vi "Read 3D Quiver  Property Array.vi"(8 "error in (no error)":errorcluster, 11 "3D Quiver.lvclass in":refnum<class "3D Quiver.lvclass">) -> (0 "error out":errorcluster, 2 "3D Quiver Property Array":T1, 3 "3D Quiver.lvclass out":refnum<class "3D Quiver.lvclass">)   [LabVIEW 2020, in "3D Quiver.lvclass"]
uses:
  <vilib>/Math Plots/3D Math Plots/3D Quiver/3D Quiver/3D Quiver.lvclass
  <vilib>/Math Plots/3D Math Plots/3D Quiver/3D Quiver/Typedef/3D Quiver Property Array.ctl
  <vilib>/Math Plots/3D Math Plots/3D Quiver/3D Quiver/Typedef/3D Quiver Property.ctl
  <vilib>/Math Plots/3D Math Plots/3D Plot/3D Plot/Typedef/Line Type.ctl
  <vilib>/Math Plots/3D Math Plots/3D Plot/3D Plot/Typedef/Color Ramp Cluster.ctl
  <vilib>/Math Plots/3D Math Plots/3D Quiver/3D Quiver/3D Quiver.lvclass/3D Quiver.ctl
  <vilib>/Math Plots/3D Math Plots/3D Plot/3D Plot/3D Plot.lvclass
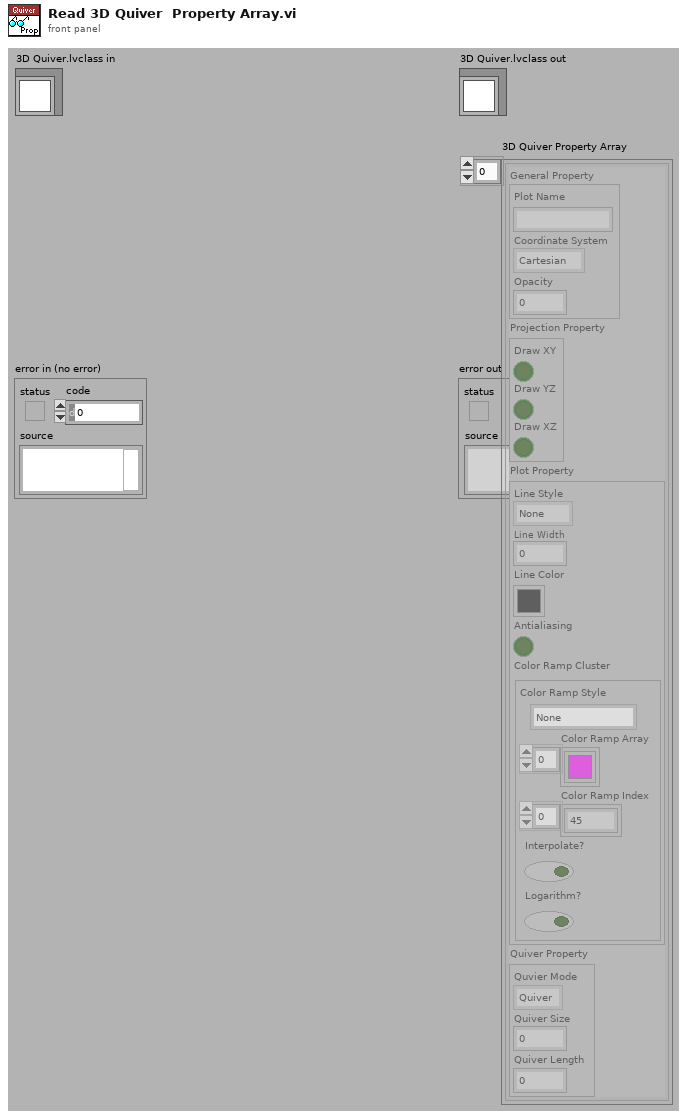
[diagram p1: front panel]
types:
  T1 = typedef "3D Quiver.lvclass/3D Quiver Property Array.ctl" = T2[]
  T2 = typedef "3D Quiver.lvclass/3D Quiver Property.ctl" = cluster{"General Property":cluster{"Plot Name":string, "Coordinate System":enum16{"Cartesian", "Cylindrical", "Spherical"}, "Opacity":sgl}, "Projection Property":cluster{"Draw XY":bool, "Draw YZ":bool, "Draw XZ":bool}, "Plot Property":cluster{"Line Style":T3, "Line Width":sgl, "Line Color":u32, "Antialiasing":bool, "Color Ramp Cluster":T4}, "Quiver Property":cluster{"Quvier Mode":enum16{"Quiver", "Quiver with surface"}, "Quiver Size":sgl, "Quiver Length":sgl}}
  T3 = typedef "3D Plot.lvclass/Line Type.ctl" = enum16{"None", "Solid", "Dash", "Dot", "Dash Dot"}
  T4 = typedef "3D Plot.lvclass/Color Ramp Cluster.ctl" = cluster{"Color Ramp Style":enum16{"None", "Shaded", "Color spectrum", "Grey scale", "Custom"}, "Color Ramp Array":u32[], "Color Ramp Index":i32[], "Interpolate?":bool, "Logarithm?":bool}
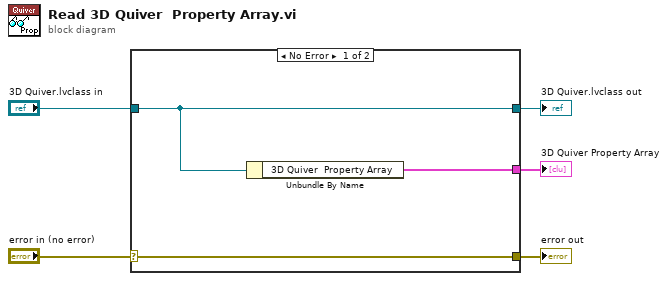
[diagram p0: block diagram]
diagram:
  n1 = case shown="No Error" "error in (no error)" {
    selector: "error in (no error)" -> [w8 w9]
    tunnel: [w8 w9] -> w4
    tunnel: [w7 w10] -> w2
    tunnel: "3D Quiver.lvclass in" -> [w7 w10]
    tunnel: [w6 _] -> w1
    frame No Error {
      n2 = Unbundle By Name(w7) -> ("3D Quiver  Property Array"=w6:T1)
    }
    frame Error {
    }
  }
  "error out" <- w4
  "3D Quiver.lvclass out" <- w2
  "3D Quiver Property Array" <- w1
